vi "Chroma 1905x Series Configure Hipot ARC Limit Query.vi"(7 "Mode":T1 items=["AC", "DC"], 8 "error in (no error)":errorcluster, 10 "Step":T2=1 min=1 max=99 step=1, 11 "VISA resource name":refnum<visa-resource-name>) -> (0 "error out":errorcluster, 3 "VISA resource name out":refnum<visa-resource-name>)   [LabVIEW 2025]
uses:
  step--control.ctl
  Type Def/modes AC DC--control.ctl
panel:
  out "ARC Limit value [A]":string
  # "ARC Limit query"
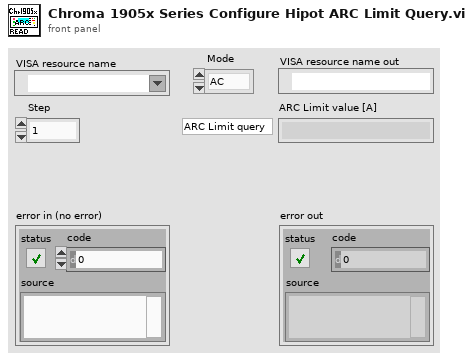
[diagram p1: front panel]
types:
  T1 = typedef "modes AC DC--control.ctl" = i32
  T2 = typedef "step--control.ctl" = u8
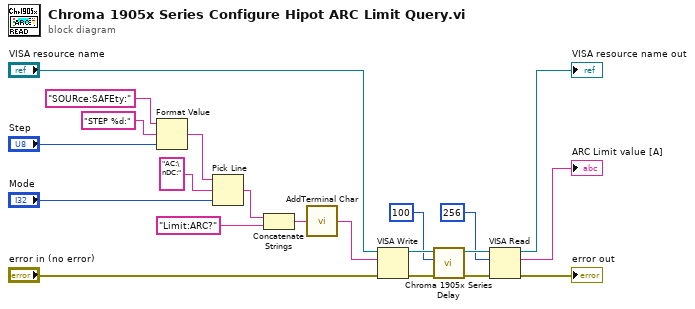
[diagram p0: block diagram]
diagram:
  n1 = Format Value(string ("")="SOURce:SAFEty:", format string="STEP %d:", value (0)="Step") -> (output string=w18:string)
  n2 = Pick Line(string ("")=w18, multi-line string="AC:\nDC:", line index="Mode") -> (output string=w14:string)
  n3 = Concatenate Strings(w14, "Limit:ARC?" ("format string")) -> (w12:string)
  n4 = call "AddTerminal Char.vi"("Cmd string"=w12) -> ("Concatenated String"=w10:string)  [unwired: 4 in]
  n5 = VISA Write(VISA resource name="VISA resource name", write buffer=w10, error in (no error)="error in (no error)") -> (VISA resource name out=w5:refnum<visa-resource-name>, error out=w7:errorcluster)  [unwired: 1 out]
  n6 = call "Chroma 1905x Series Delay.vi"("error in (no error)"=w7, "Time Delay [ms]"=u32 100 ("Time Delay ms"), "VISA resource name"=w5) -> ("error out"=w6:errorcluster, "VISA resource name 2"=w4:refnum<visa-resource-name>)  [unwired: 7 in]
  n7 = VISA Read(VISA resource name=w4, byte count=u32 256, error in (no error)=w6) -> (VISA resource name out=→"VISA resource name out":refnum<visa-resource-name>, read buffer=→"ARC Limit value [A]":string, error out=→"error out":errorcluster)  [unwired: 1 out]
